vi "Query Time.vi"(8 "error IO":errorcluster, 11 "VISA resource name":refnum<visa-resource-name>) -> (0 "error Out":errorcluster, 1 "Minute":i32 format="%02d", 2 "Hour":i32 format="%02d", 3 "VISA resource Out":refnum<visa-resource-name>)   [LabVIEW 2016, in "eec EST 300.lvlib"]
doc: "Returns the system time. Results will be returned as 2 digit integers. If 24 hour format is enabled the PM? boolean will always be false."
uses:
  <instrlib>/eec EST 300/eec EST 300.lvlib
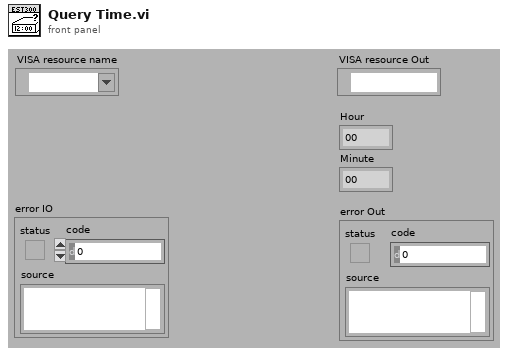
[diagram p1: front panel]
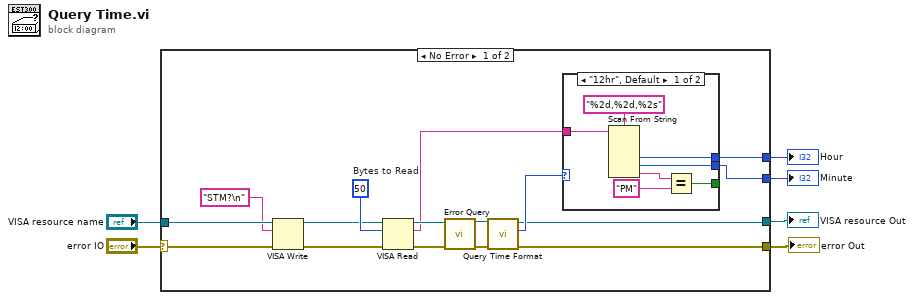
[diagram p0: block diagram]
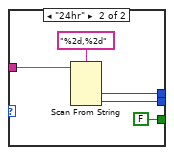
[diagram p2: hidden frame]
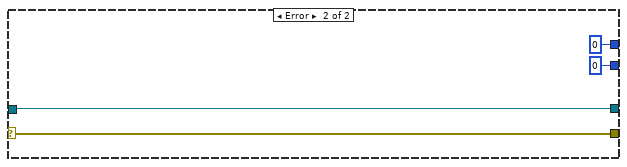
[diagram p3: hidden frame]
diagram:
  n1 = case shown="No Error" "error IO" {
    selector: "error IO" -> [w22 w38]
    tunnel: [w10 w38] -> w3
    tunnel: [w11 w37] -> w4
    tunnel: "VISA resource name" -> [w21 w37]
    tunnel: [w9 0] -> w2
    tunnel: [w8 0] -> w1
    frame No Error {
      w19 = u32 50  # Bytes to Read
      n2 = VISA Write(VISA resource name=w21, write buffer="STM?\n" ("Command to Send (empty)"), error in (no error)=w22) -> (VISA resource name out=w16:refnum<visa-resource-name>, error out=w15:errorcluster)  [unwired: 1 out]
      n3 = VISA Read(VISA resource name=w16, byte count=w19, error in (no error)=w15) -> (VISA resource name out=w18:refnum<visa-resource-name>, read buffer=w7:string, error out=w17:errorcluster)  [unwired: 1 out]
      n4 = call <instrlib>:"Error Query.vi"("VISA resource name"=w18, "error in (no error)"=w17) -> ("VISA resource name out"=w13:refnum<visa-resource-name>, "error out"=w14:errorcluster)  [unwired: 10 in, 2 out]
      n5 = call <instrlib>:"Query Time Format.vi"("error IO"=w14, "VISA resource name"=w13) -> ("error Out"=w10:errorcluster, "Time Format"=w12:enum16{"12hr", "24hr"}, "VISA resource Out"=w11:refnum<visa-resource-name>)  [unwired: 7 in]
      n6 = case shown="\"12hr\", Default" w12 {
        tunnel: w7 -> [w28 w33]
        tunnel: [w27 w32] -> w9
        tunnel: [w26 w31] -> w8
        tunnel: [w23 FALSE] -> _
        frame "12hr", Default {
          n7 = Scan From String(format string="%2d,%2d,%2s", input string=w28) -> (output 1=w27:i32, output 2=w26:i32, output 3=w25:string)  [unwired: 5 in, 3 out]
          n8 = Equal?(x=w25, y="PM") -> (x = y?=w23:bool)
        }
        frame "24hr" {
          n9 = Scan From String(format string="%2d,%2d", input string=w33) -> (output 1=w32:i32, output 2=w31:i32)  [unwired: 4 in, 3 out]
        }
      }
    }
    frame Error {
    }
  }
  "VISA resource Out" <- w4
  "error Out" <- w3
  "Hour" <- w2
  "Minute" <- w1
